vi "Populate CAN Interface Name Menu.vi"(8 "error in":errorcluster, 11 "CAN Interface Menu Refnum":refnum<vi>) -> (0 "error out":errorcluster)   [LabVIEW 2020, in "Communication Bus Template System Explorer.lvlib" / "Implementation.lvlib"]
uses:
  Implementation.lvlib
  <vilib>/Utility/miscctls.llb/LVStringsAndValuesArrayTypeDef_U16.ctl
  Types/XNET Interface Name.ctl
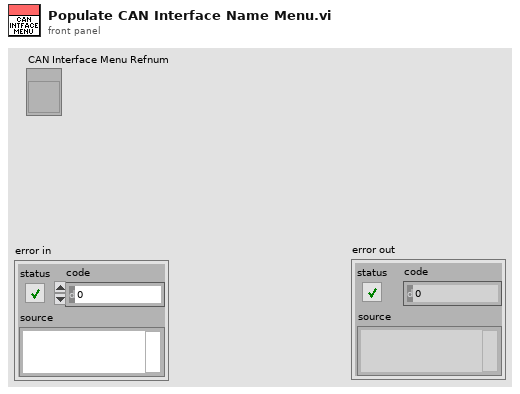
[diagram p1: front panel]
types:
  T1 = typedef "LVStringsAndValuesArrayTypeDef_U16.ctl" = cluster{"String":string, "Value":u16}[]
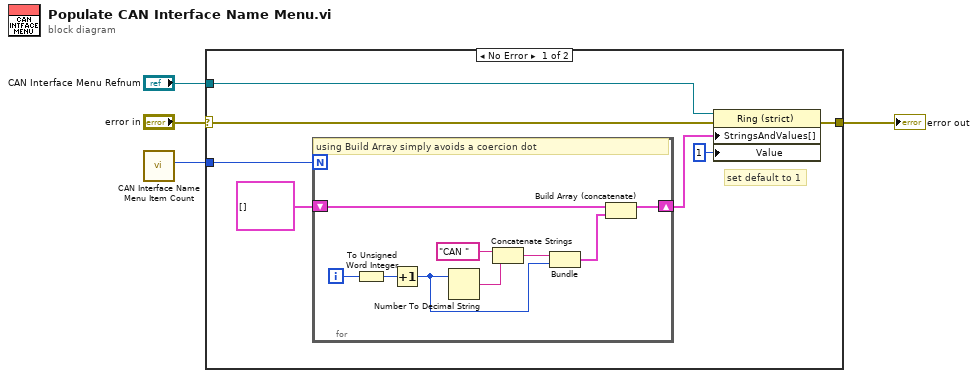
[diagram p0: block diagram]
diagram:
  n1 = call "CAN Interface Name Menu Item Count.vi"() -> ("number of menu items"=w1:u16)  [unwired: 11 in]
  n2 = case shown="No Error" "error in" {
    selector: "error in" -> [w9 w21]
    tunnel: w1 -> [w11 _]
    tunnel: "CAN Interface Menu Refnum" -> [w10 _]
    tunnel: [w8 w21] -> w2
    frame No Error {
      # "set default to 1"
      n3 = for {
        N: w11 -> [_]
        shift-right: [w12] -> w6
        shift-left: T1 [] ("Strings And Values []") -> [w14]
        i -> [w20]
        # "using Build Array simply avoids a coercion dot"
        n4 = To Unsigned Word Integer(number=w20) -> (unsigned 16bit integer=w19:u16)
        n5 = Increment(x=w19) -> (x+1=w15:u16)
        n6 = Number To Decimal String(number=w15) -> (decimal integer string=w17:string)  [unwired: 1 in]
        n7 = Concatenate Strings("CAN ", w17) -> (w16:string)
        n8 = Bundle(w16, w15) -> (w13:cluster{string, u16})  [unwired: 1 in]
        n9 = Build Array (concatenate)(w14, w13) -> (w12:T1)
      }
      n10 = property class="Ring (strict)"(reference=w10, error in=w9, "StringsAndValues[]"=w6, "Value"=u16 1) -> (error out=w8:errorcluster)  [unwired: 1 out]
    }
    frame Error {
    }
  }
  "error out" <- w2
